vi "HexapodHardwareMove.vi"(7 "xyzuvw":dbl[](array[numeric]), 8 "error in (no error)":errorcluster, 9 "Positions of Axes to move":dbl[](array[numeric]), 10 "Axes to move":string[](array[string]), 11 "HexapodPI in":refnum<class "HexapodPI.lvclass">) -> (0 "error out":errorcluster, 2 "Connection":T1, 3 "Move possible":cluster{"status":bool, "message":string})   [LabVIEW 2020, in "HexapodPI.lvclass"]
uses:
  HexapodPI.lvclass
  HexapodPI.lvclass/HexapodPI.ctl
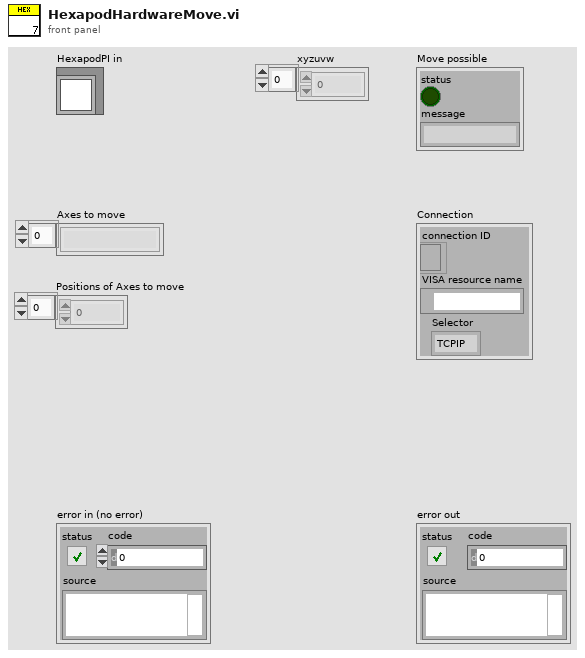
[diagram p1: front panel]
types:
  T1 = cluster{"connection ID":refnum<k5>, "VISA resource name":refnum<visa-resource-name>, "Selector":enum16{"TCPIP", "Serial"}}
  T2 = typedef "OnOffTypeDef.ctl" = enum16{"off", "on"}
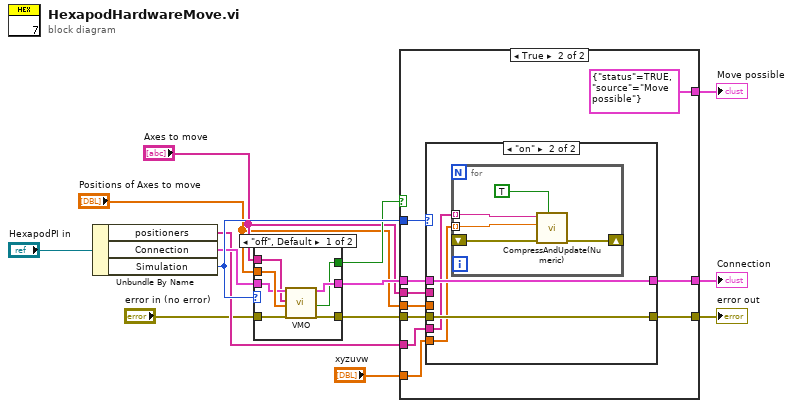
[diagram p0: block diagram]
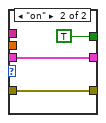
[diagram p2: hidden frame]
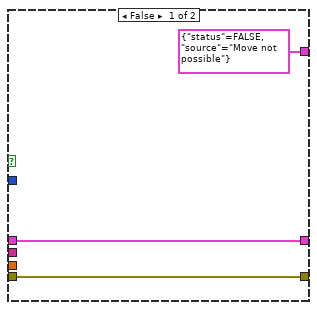
[diagram p3: hidden frame]
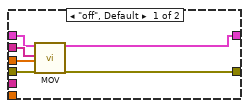
[diagram p4: hidden frame]
diagram:
  n1 = Unbundle By Name("HexapodPI in") -> ("positioners"=w11:string[], "Connection"=w12:T1, "Simulation"=w13:T2)
  n2 = case shown="\"off\", Default" w13 {
    tunnel: "error in (no error)" -> [w21 w22]
    tunnel: "Positions of Axes to move" -> [w20 _]
    tunnel: w12 -> [w19 w24]
    tunnel: "Axes to move" -> [w18 _]
    tunnel: [w17 w24] -> w5
    tunnel: [w16 w22] -> w6
    tunnel: [w15 TRUE ("Move possible")] -> w8
    frame "off", Default {
      n3 = call "VMO.vi"("Connection"=w19, "Axes to command"=w18, "Position values"=w20, "error in"=w21) -> ("Connection out"=w17:T1, "Move possible"=w15:bool, "error out"=w16:errorcluster)  [unwired: 13 in]
    }
    frame "on" {
    }
  }
  n4 = case shown="True" w8 {
    tunnel: w6 -> [w26 w37]
    tunnel: [w26 w36] -> w2
    tunnel: "Axes to move" -> [_ w35]
    tunnel: "Positions of Axes to move" -> [_ w34]
    tunnel: w5 -> [w27 w33]
    tunnel: [w27 w32] -> w9
    tunnel: [cluster{"status":bool, "source":string} {"status"=FALSE, "source"="Move not possible"} ("error out") cluster{"status":bool, "source":string} {"status"=TRUE, "source"="Move possible"} ("error out")] -> w7
    tunnel: w13 -> [_ w30]
    tunnel: w11 -> [_ w29]
    tunnel: "xyzuvw" -> [_ w28]
    frame False {
    }
    frame True {
      n5 = case shown="\"on\"" w30 {
        tunnel: w37 -> [w43 w46]
        tunnel: [w42 w46] -> w36
        tunnel: w35 -> [w41 _]
        tunnel: w34 -> [w40 _]
        tunnel: w33 -> [w39 w47]
        tunnel: [w38 w47] -> w32
        tunnel: w29 -> [_ w45]
        tunnel: w28 -> [_ w44]
        frame "off", Default {
          n6 = call "MOV.vi"("Connection"=w39, "Axes to move"=w41, "Position values"=w40, "error in"=w43) -> ("Connection out"=w38:T1, "error out"=w42:errorcluster)  [unwired: 14 in]
        }
        frame "on" {
          n7 = for {
            tunnel: w45 -> [w49] mode=indexing
            shift-right: [w52] -> _
            shift-left: _ -> [w50]
            tunnel: w44 -> [w48] mode=indexing
            n8 = call "CompressAndUpdate(Numeric).vi"("force CVT update (false)"=TRUE, "error in"=w50, "Numeric"=w48, "command or variable name"=w49) -> ("error out"=w52:errorcluster)  [unwired: 7 in]
          }
        }
      }
    }
  }
  "Connection" <- w9
  "Move possible" <- w7
  "error out" <- w2
